vi "Read.vi"(8 "Error In":errorcluster, 10 "UART Channel (0)":u8, 11 "LINX Resource":T1) -> (0 "Error Out":errorcluster, 2 "Distance (in)":u32, 3 "LINX Resource":T1)   [LabVIEW 2020, in "LMH-LINX.lvlib" / "PmodMAXSONAR.lvlib"]
doc: "Read distance in inches from the PmodMAXSONAR."
uses:
  PmodMAXSONAR.lvlib
  Private/Type Defs/LINX Ref.ctl
  Private/Type Defs/Platform.ctl
  Private/Type Defs/Interface.ctl
  Private/Device/Type Defs/LINX Device Config.ctl
  Private/Device/Type Defs/TCP Config.ctl
  Private/Device/Type Defs/Channels.ctl
  Peripherals/UART/UART Read String.vi
  LMH-LINX.lvlib
  Private/Device/Device.lvlib
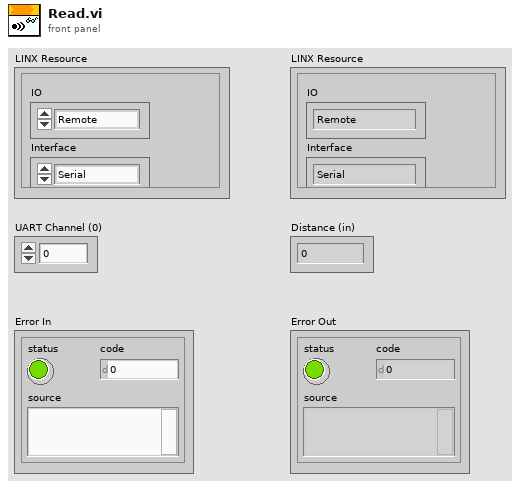
[diagram p1: front panel]
types:
  T1 = typedef "LMH-LINX.lvlib/LINX Ref.ctl" = cluster{"IO":T2, "Interface":T3, "LINX Device Config":T4}
  T2 = typedef "LMH-LINX.lvlib/Platform.ctl" = enum16{"Remote", "Local"}
  T3 = typedef "LMH-LINX.lvlib/Interface.ctl" = enum16{"Serial", "TCP"}
  T4 = typedef "Device.lvlib/LINX Device Config.ctl" = cluster{"Interface":T3, "COM Port":refnum<visa-resource-name>, "TCP Configuration":T5, "Device Family":u8, "Device ID":u8, "Device Name":string, "TCP Ref":refnum<k5>, "Channels":T6}
  T5 = typedef "Device.lvlib/TCP Config.ctl" = cluster{"IP Address":string, "Port":u16}
  T6 = typedef "LMH-LINX.lvlib/Channels.ctl" = cluster{"DI":u8[], "DO":u8[], "AI":u8[], "AO":u8[], "PWM":u8[], "QE":u8[], "UART":u8[], "I2C 2":u8[], "SPI":u8[], "CAN":u8[], "Servo":u8[], "AI Ref (V)":dbl, "AI Resolution (Bits)":u8, "AO Ref (V)":dbl, "AO Resolution (Bits)":u8}
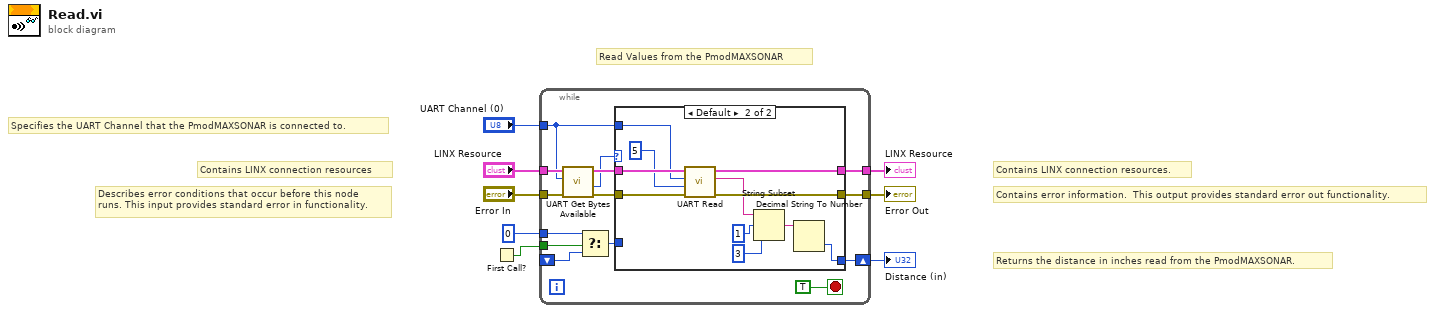
[diagram p0: block diagram]
diagram:
  # "Read Values from the PmodMAXSONAR"
  # "Returns the distance in inches read from the PmodMAXSONAR."
  # "Contains error information.  This output provides standard error out functionality."
  # "Contains LINX connection resources."
  # "Describes error conditions that occur before this node\nruns. This input provides standard error in functionality."
  # "Contains LINX connection resources"
  # "Specifies the UART Channel that the PmodMAXSONAR is connected to."
  n1 = First Call?() -> (First Call?: T/F=w4:bool)
  n2 = while {
    tunnel: [w21] -> w6
    tunnel: [w22] -> w8
    tunnel: "UART Channel (0)" -> [w12]
    shift-right: [w20] -> w5
    shift-left: _ -> [w18]
    tunnel: w4 -> [w17]
    tunnel: 0 -> [w16]
    tunnel: "Error In" -> [w14]
    tunnel: "LINX Resource" -> [w13]
    stop <- TRUE stop-if-true
    n3 = call "UART Get Bytes Available.vi"("Error In"=w14, "UART Channel (0)"=w12, "LINX Resource"=w13) -> ("Error Out"=w10:errorcluster, "Bytes Available"=w9:u8, "LINX Resource"=w11:T1)  [unwired: 6 in]
    n4 = Select(t=w16, s=w17, f=w18) -> (s? t:f=w15:i32)
    n5 = case shown="Default" w9 {
      tunnel: w11 -> [w25 w36]
      tunnel: w10 -> [w24 w35]
      tunnel: [w25 w34] -> w21
      tunnel: [w24 w33] -> w22
      tunnel: w12 -> [_ w31]
      tunnel: [w23 w27] -> w20
      tunnel: w15 -> [w23 _]
      frame 0 {
      }
      frame Default {
        n6 = call-poly "UART Read.vi"("Error In"=w35, "Num Bytes"=u8 5, "UART Channel (0)"=w31, "LINX Resource"=w36) -> ("Error Out"=w33:errorcluster, "Data"=w26:string, "LINX Resource"=w34:T1)  [unwired: 5 in]
        n7 = String Subset(string=w26, offset (0)=1, length (rest)=3 ("length (rest)")) -> (substring=w28:string)
        n8 = Decimal String To Number(string=w28) -> (number=w27:i32)  [unwired: 2 in, 1 out]
      }
    }
  }
  "Error Out" <- w8
  "LINX Resource" <- w6
  "Distance (in)" <- w5
